vi "Auto Setup Osciloscope.vi"(8 "error in (no error)":errorcluster, 11 "Tektronicks in":refnum<class "Tektronicks.lvclass">) -> (0 "error out":errorcluster, 3 "Tektronicks out":refnum<class "Tektronicks.lvclass">)   [LabVIEW 2020, in "Tektronicks.lvclass"]
uses:
  Tektronicks.lvclass
  Tektronicks.lvclass/Tektronicks.ctl
  <instrlib>/Tektronix TDS 200 1000 2000 Series/Tektronix TDS 200 1000 2000 Series.lvlib
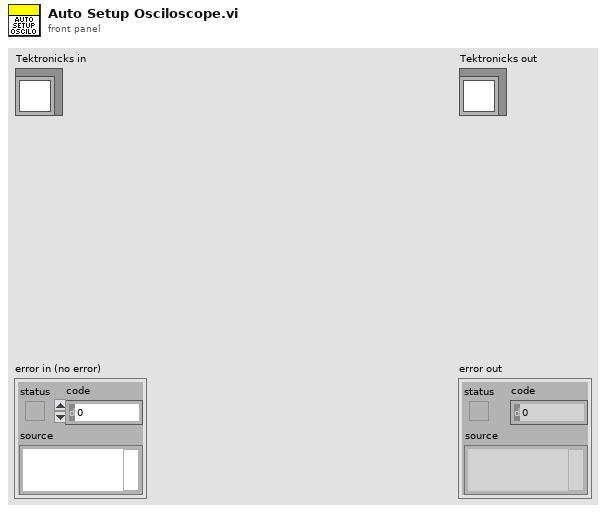
[diagram p1: front panel]
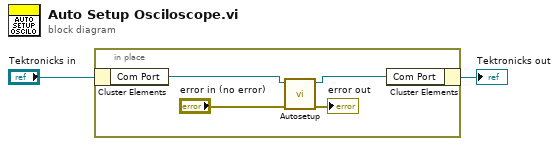
[diagram p0: block diagram]
diagram:
  n1 = in-place {
    n2 = in-place-cluster #1("Tektronicks in") -> ("Com Port"=w4:refnum<visa-resource-name>)
    n3 = call <instrlib>:"Autosetup.vi"("error in (no error)"="error in (no error)", "VISA resource name"=w4) -> ("error out"=→"error out":errorcluster, "VISA resource name out"=w3:refnum<visa-resource-name>)  [unwired: 8 in]
    n4 = in-place-cluster #1("Com Port"=w3) -> (→"Tektronicks out":refnum<class "Tektronicks.lvclass">)
  }
